vi "bundle JSON& bindata to Bindata&descr cluster.vi"(8 "error in (no error)":errorcluster, 9 "name":string="img", 10 "binary data received":u8[](array[numeric]), 11 "JSON received":string) -> (0 "error out":errorcluster, 2 "index":i32, 3 "Bindata & descr out":T1)   [LabVIEW 2018, in "LV2Julia_core.lvlib"]
doc: "Takes data received from Julia server - JSON and binary. From these select a subset by the name provided to the name input and bundle the data to a cluster for the further processing by LabView, e.g. to a numeric array or an image."
uses:
  LV2Julia_core.lvlib
  Bindata&description.ctl
  Bindata description.ctl
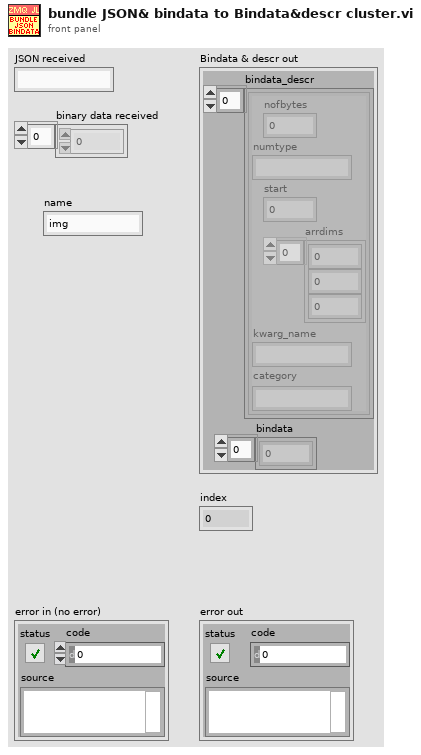
[diagram p1: front panel]
types:
  T1 = typedef "LV2Julia_core.lvlib/Bindata&description.ctl" = cluster{"bindata_descr":T2[], "bindata":u8[]}
  T2 = typedef "LV2Julia_core.lvlib/Bindata description.ctl" = cluster{"nofbytes":i32, "numtype":string, "start":i32, "arrdims":i32[], "kwarg_name":string, "category":string}
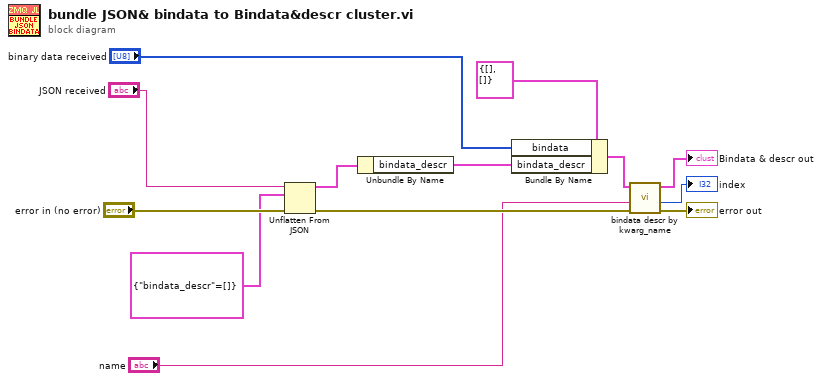
[diagram p0: block diagram]
diagram:
  n1 = Unflatten From JSON(JSON string="JSON received", type and defaults=cluster{"bindata_descr":T2[]} {"bindata_descr"=[]}, error in (no error)="error in (no error)") -> (value=w7:cluster{"bindata_descr":T2[]}, error out=w10:errorcluster)  [unwired: 4 in]
  n2 = Unbundle By Name(w7) -> ("bindata_descr"=w8:T2[])
  n3 = Bundle By Name(cluster=T1 {"bindata_descr"=[], "bindata"=[]} ("Bindata & descr"), "bindata"="binary data received", "bindata_descr"=w8) -> (w1:T1)
  n4 = call "bindata descr by kwarg_name.vi"("Error in"=w10, "kwarg_name"="name", "Bindata & descr"=w1) -> ("Error out"=→"error out":errorcluster, "index"=→"index":i32, "Bindata & descr out"=→"Bindata & descr out":T1)  [unwired: 5 in, 1 out]
